vi "更新因子配置.vi"(8 "error in (no error)":errorcluster caption="错误输入（无错误）") -> (0 "error out":errorcluster caption="错误输出")   [LabVIEW 2016, in "数据传输系统.lvlib"]
uses:
  <vilib>/Utility/config.llb/Read Key (String).vi
  <vilib>/Utility/config.llb/Write Key (String).vi
  <vilib>/Utility/config.llb/Write Key (Boolean).vi
  <vilib>/Utility/config.llb/NI_LVConfig.lvlib
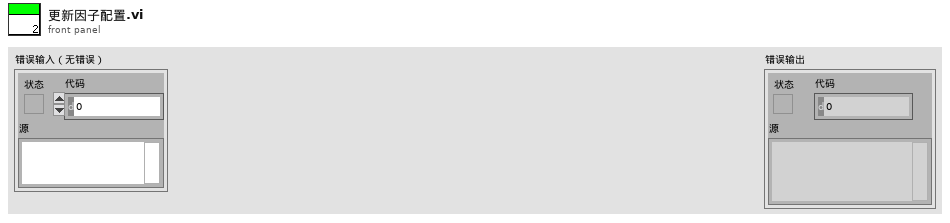
[diagram p1: front panel]
types:
  T1 = cluster{"setini":string, "sysini":string, "hechaini":string, "actualwrite":string, "actualread":string, "datasent":string, "反控命令信息队列":string, "反控与仪器交互":string}
  T2 = typedef "NI_LVConfig.lvlib/Config Data RefNum.ctl" = refnum<k1>
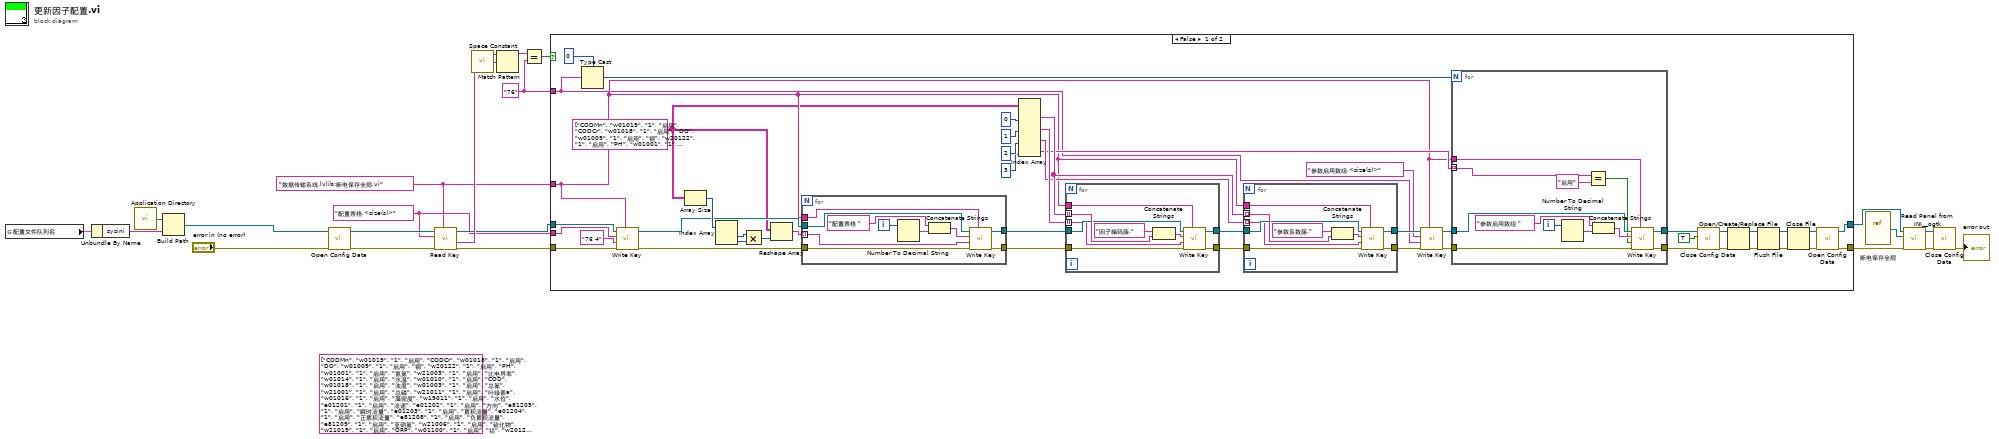
[diagram p0: block diagram]
diagram:
  (unwired) string[][] [["CODMn", "w01019", "1", "启用"], ["CODCr", "w01018", "1", "启用"], ["DO", "w01009", "1", "启用"], ["铜", "w20122", "1", "启用"], ["PH", "w01001", "1", "启用"], ["氨氮", "w21003", "1", "启用"], ["比电导率", "w01014", "1", "启用"], ["水温", "w01010", "1", "启用"], ["COD", "w01018", "1", "启用"], ["浊度", "w01003", "1", "启用"], ["总氮", "w21001", "1", "启用"], ["总磷", "w21011", "1", "启用"], ["叶绿素a", "w01016", "1", "启用"], ["藻密度", "w19011", "1", "启用"], ["水位", "e01201", "1", "启用"], ["流速", "e01202", "1", "启用"], ["方向", "e81205", "1", "启用"], ["瞬时流量", "e01203", "1", "启用"], ["累积流量", "e01204", "1", "启用"], ["正累积流量", "e81208", "1", "启用"], ["负累积流量", "e81209", "1", "启用"], ["亚硝氮", "w21006", "1", "启用"], ["硫化物", "w21019", "1", "启用"], ["ORP", "w01100", "1", "启用"], ["铅", "w20120", "1", "启用"], ["镉", "w20115", "1", "启用"], ["锌", "w20123", "1", "启用"], ["镍", "w20121", "1", "启用"], ["锰", "w20124", "1", "启用"], ["汞", "w20111", "1", "启用"], ["气温", "a01001", "1", "启用"], ["气压", "e01901", "1", "启用"], ["风速", "e01301", "1", "启用"], ["风向", "e01302", "1", "启用"], ["空气温度", "e01001", "1", "启用"], ["相对湿度", "e01002", "1", "启用"], ["分钟雨量", "e01303", "1", "启用"], ["小时雨量", "e013031", "1", "启用"], ["日雨量", "e013032", "1", "启用"], ["累积雨量", "e013033", "1", "启用"], ["盐度", "w01002", "1", "启用"], ["磷酸盐", "w21015", "1", "启用"], ["硝氮", "w21007", "1", "启用"], ["氟化物", "w21017", "1", "启用"], ["挥发酚", "w23002", "1", "启用"], ["氯化物", "w21002", "1", "启用"], ["蓝绿藻", "w01022", "1", "启用"], ["余氯", "w21012", "1", "启用"], ["综合生物毒性", "w01023", "1", "启用"], ["艏向", "e81216", "1", "启用"], ["横摇", "e81217", "1", "启用"], ["纵摇", "e81218", "1", "启用"], ["分层标志", "e81220", "1", "启用"], ["层状态1", "e81221", "1", "启用"], ["层状态2", "e81222", "1", "启用"], ["水平平均流速", "e81225", "1", "启用"], ["流向", "e80015", "1", "启用"], ["北向流速分量", "e81223", "1", "启用"], ["东向流速分量", "e81224", "1", "启用"], ["垂直流速分量", "e81219", "1", "启用"], ["最大波高", "e80001", "1", "启用"], ["最大波周期", "e80002", "1", "启用"], ["1/10波高", "e80003", "1", "启用"], ["1/10波周期", "e80004", "1", "启用"], ["有效波高", "e80005", "1", "启用"], ["有效波周期", "e80006", "1", "启用"], ["平均波高", "e80007", "1", "启用"], ["平均波周期", "e80008", "1", "启用"], ["波向", "e80009", "1", "启用"], ["波个数", "e80016", "1", "启用"], ["水深", "e81231", "1", "启用"], ["X轴流速", "e81226", "1", "启用"], ["Y轴流速", "e81227", "1", "启用"], ["信号强度", "e81228", "1", "启用"], ["电压", "e81215", "1", "启用"]] ("配置表格")
  w12 = "76" ("y")
  w14 = "配置表格.<size(s)>" ("key")
  w13 = "数据传输系统.lvlib:断电保存全局.vi" ("section")
  n1 = global read "全局1.vi" "配置文件队列名"() -> (w20:T1)
  n2 = Unbundle By Name(w20) -> ("sysini"=w22:string)
  n3 = call <vilib>:"Application Directory.vi"() -> ("Application Directory"=w21:path)
  n4 = Build Path(base path=w21, name or relative path=w22) -> (appended path=w9:path)
  n5 = call <vilib>:"Open Config Data.vi"("error in (no error)"="error in (no error)", "configuration file path"=w9) -> ("error out"=w5:errorcluster, "refnum"=w19:T2)  [unwired: 7 in, 1 out]
  n6 = call-poly <vilib>:"Read Key.vi"("section"=w13, "error in (no error)"=w5, "key"=w14, "refnum"=w19) -> ("error out"=w10:errorcluster, "value"=w18:string, "refnum out"=w15:T2)  [unwired: 4 in, 1 out]
  n7 = call <vilib>:"Space Constant.vi"() -> ("String"=w17:string)
  n8 = Match Pattern(string=w18, regular expression=w17) -> (before substring=w16:string)  [unwired: 1 in, 3 out]
  n9 = Equal?(x=w16, y=w12) -> (x = y?=w11:bool)
  n10 = case shown="False" w11 {
    tunnel: w15 -> [w38 w110]
    tunnel: w14 -> [w63 _]
    tunnel: w13 -> [w45 _]
    tunnel: w12 -> [w42 _]
    tunnel: w10 -> [w37 w109]
    tunnel: [w25 w110] -> w2
    tunnel: [w24 w109] -> w1
    frame False {
      w23 = string[][] [["CODMn", "w01019", "1", "启用"], ["CODCr", "w01018", "1", "启用"], ["DO", "w01009", "1", "启用"], ["铜", "w20122", "1", "启用"], ["PH", "w01001", "1", "启用"], ["氨氮", "w21003", "1", "启用"], ["比电导率", "w01014", "1", "启用"], ["水温", "w01010", "1", "启用"], ["COD", "w01018", "1", "启用"], ["浊度", "w01003", "1", "启用"], ["总氮", "w21001", "1", "启用"], ["总磷", "w21011", "1", "启用"], ["叶绿素a", "w01016", "1", "启用"], ["藻密度", "w19011", "1", "启用"], ["水位", "e01201", "1", "启用"], ["流速", "e01202", "1", "启用"], ["方向", "e81205", "1", "启用"], ["瞬时流量", "e01203", "1", "启用"], ["累积流量", "e01204", "1", "启用"], ["正累积流量", "e81208", "1", "启用"], ["负累积流量", "e81209", "1", "启用"], ["亚硝氮", "w21006", "1", "启用"], ["硫化物", "w21019", "1", "启用"], ["ORP", "w01100", "1", "启用"], ["铅", "w20120", "1", "启用"], ["镉", "w20115", "1", "启用"], ["锌", "w20123", "1", "启用"], ["镍", "w20121", "1", "启用"], ["锰", "w20124", "1", "启用"], ["汞", "w20111", "1", "启用"], ["气温", "a01001", "1", "启用"], ["气压", "e01901", "1", "启用"], ["风速", "e01301", "1", "启用"], ["风向", "e01302", "1", "启用"], ["空气温度", "e01001", "1", "启用"], ["相对湿度", "e01002", "1", "启用"], ["分钟雨量", "e01303", "1", "启用"], ["小时雨量", "e013031", "1", "启用"], ["日雨量", "e013032", "1", "启用"], ["累积雨量", "e013033", "1", "启用"], ["盐度", "w01002", "1", "启用"], ["磷酸盐", "w21015", "1", "启用"], ["硝氮", "w21007", "1", "启用"], ["氟化物", "w21017", "1", "启用"], ["挥发酚", "w23002", "1", "启用"], ["氯化物", "w21002", "1", "启用"], ["蓝绿藻", "w01022", "1", "启用"], ["余氯", "w21012", "1", "启用"], ["综合生物毒性", "w01023", "1", "启用"], ["艏向", "e81216", "1", "启用"], ["横摇", "e81217", "1", "启用"], ["纵摇", "e81218", "1", "启用"], ["分层标志", "e81220", "1", "启用"], ["层状态1", "e81221", "1", "启用"], ["层状态2", "e81222", "1", "启用"], ["水平平均流速", "e81225", "1", "启用"], ["流向", "e80015", "1", "启用"], ["北向流速分量", "e81223", "1", "启用"], ["东向流速分量", "e81224", "1", "启用"], ["垂直流速分量", "e81219", "1", "启用"], ["最大波高", "e80001", "1", "启用"], ["最大波周期", "e80002", "1", "启用"], ["1/10波高", "e80003", "1", "启用"], ["1/10波周期", "e80004", "1", "启用"], ["有效波高", "e80005", "1", "启用"], ["有效波周期", "e80006", "1", "启用"], ["平均波高", "e80007", "1", "启用"], ["平均波周期", "e80008", "1", "启用"], ["波向", "e80009", "1", "启用"], ["波个数", "e80016", "1", "启用"], ["水深", "e81231", "1", "启用"], ["X轴流速", "e81226", "1", "启用"], ["Y轴流速", "e81227", "1", "启用"], ["信号强度", "e81228", "1", "启用"], ["电压", "e81215", "1", "启用"], ["悬浮物", "w01012", "1", "启用"]] ("配置表格")
      n11 = Type Cast(type=0, x=w42) -> (*(type *) &x=w47:i32)
      n12 = call-poly <vilib>:"Write Key.vi"("section"=w45, "error in (no error)"=w37, "value"="76 4" ("y"), "key"=w63, "refnum"=w38) -> ("error out"=w60:errorcluster, "refnum out"=w61:T2)  [unwired: 4 in, 1 out]
      n13 = Array Size(array=w23) -> (size(s)=w68:i32[])
      n14 = Index Array(array=w68) -> (element #1=w66:i32, element #2=w67:i32)  [unwired: 2 in]
      n15 = Multiply(x=w66, y=w67) -> (x*y=w65:i32)
      n16 = Reshape Array(w23, w65) -> (w62:string[])
      n17 = for {
        tunnel: w62 -> [w104] mode=indexing
        tunnel: w45 -> [w103]
        tunnel: w61 -> [w102]
        tunnel: w60 -> [w101]
        tunnel: [w100] -> w58
        tunnel: [w99] -> w57
        i -> [w108]
        n18 = Number To Decimal String(number=w108) -> (decimal integer string=w107:string)  [unwired: 1 in]
        n19 = Concatenate Strings("配置表格 ", w107) -> (w105:string)
        n20 = call-poly <vilib>:"Write Key.vi"("section"=w103, "error in (no error)"=w101, "value"=w104, "key"=w105, "refnum"=w102) -> ("error out"=w99:errorcluster, "refnum out"=w100:T2)  [unwired: 4 in, 1 out]
      }
      n21 = Index Array(array=w23, index (col) #1=0 ("禁用的索引 (列)"), index (col) #2=1 ("索引 (列)"), index (col) #3=2 ("索引 (列)"), index (col) #4=3 ("索引 (列)")) -> (element #1=w50:string[], element #2=w55:string[], element #3=w49:string[], element #4=w46:string[])  [unwired: 4 in]
      n22 = for {
        tunnel: w50 -> [w97] mode=indexing
        tunnel: w58 -> [w96]
        tunnel: w57 -> [w95]
        tunnel: w45 -> [w94]
        tunnel: w55 -> [w92] mode=indexing
        tunnel: [w91] -> w54
        tunnel: [w90] -> w53
        n23 = Concatenate Strings("因子编码簇.", w97) -> (w93:string)
        n24 = call-poly <vilib>:"Write Key.vi"("section"=w94, "error in (no error)"=w95, "value"=w92, "key"=w93, "refnum"=w96) -> ("error out"=w90:errorcluster, "refnum out"=w91:T2)  [unwired: 4 in, 1 out]
      }
      n25 = for {
        tunnel: w50 -> [w88] mode=indexing
        tunnel: w54 -> [w87]
        tunnel: w53 -> [w86]
        tunnel: w45 -> [w85]
        tunnel: w49 -> [w83] mode=indexing
        tunnel: [w82] -> w44
        tunnel: [w81] -> w40
        n26 = Concatenate Strings("参数系数簇.", w88) -> (w84:string)
        n27 = call-poly <vilib>:"Write Key.vi"("section"=w85, "error in (no error)"=w86, "value"=w83, "key"=w84, "refnum"=w87) -> ("error out"=w81:errorcluster, "refnum out"=w82:T2)  [unwired: 4 in, 1 out]
      }
      n28 = call-poly <vilib>:"Write Key.vi"("section"=w45, "error in (no error)"=w40, "value"=w42, "key"="参数启用数组.<size(s)>", "refnum"=w44) -> ("error out"=w39:errorcluster, "refnum out"=w41:T2)  [unwired: 4 in, 1 out]
      n29 = for {
        N: w47 -> [_]
        tunnel: w41 -> [w80]
        tunnel: w39 -> [w79]
        tunnel: w45 -> [w78]
        tunnel: w46 -> [w71] mode=indexing
        tunnel: [w73] -> w27
        tunnel: [w72] -> w26
        i -> [w77]
        n30 = Number To Decimal String(number=w77) -> (decimal integer string=w75:string)  [unwired: 1 in]
        n31 = Equal?(x=w71, y="启用") -> (x = y?=w69:bool)
        n32 = Concatenate Strings("参数启用数组 ", w75) -> (w74:string)
        n33 = call-poly <vilib>:"Write Key.vi"("section"=w78, "error in (no error)"=w79, "value"=w69, "key"=w74, "refnum"=w80) -> ("error out"=w72:errorcluster, "refnum out"=w73:T2)  [unwired: 4 in, 1 out]
      }
      n34 = call <vilib>:"Close Config Data.vi"("error in (no error)"=w26, "write file if changed (T)"=TRUE, "refnum"=w27) -> ("error out"=w34:errorcluster, "file path"=w33:path)  [unwired: 7 in]
      n35 = Open/Create/Replace File(file path (use dialog)=w33, error in=w34) -> (refnum out=w30:refnum<file>, error out=w31:errorcluster)  [unwired: 4 in, 1 out]
      n36 = Flush File(refnum=w30, error in=w31) -> (refnum out=w29:refnum<file>, error out=w28:errorcluster)
      n37 = Close File(refnum=w29, error in=w28) -> (path=w35:path, error out=w36:errorcluster)
      n38 = call <vilib>:"Open Config Data.vi"("error in (no error)"=w36, "configuration file path"=w35) -> ("error out"=w24:errorcluster, "refnum"=w25:T2)  [unwired: 7 in, 1 out]
    }
    frame True {
    }
  }
  n39 = vi-ref "断电保存全局.vi"() -> (w6:refnum<vi>)
  n40 = call <userlib>:"Read Panel from INI__ogtk.vi"("error in (no error)"=w1, "VI ref"=w6, "refnum"=w2) -> ("error out"=w8:errorcluster, "refnum out"=w7:T2)  [unwired: 7 in]
  n41 = call <vilib>:"Close Config Data.vi"("error in (no error)"=w8, "refnum"=w7) -> ("error out"=→"error out":errorcluster)  [unwired: 8 in, 1 out]
